vi "3phColor.vi"(4 "error in (no error)":errorcluster, 7 "Waveform Graph":refnum<vi>) -> (0 "error out":errorcluster)   [LabVIEW 2010]
panel:
  out "Array":u32[](array[numeric]) format="%06x"
  out "Label.Text":string
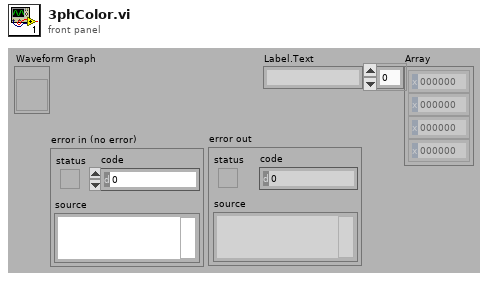
[diagram p1: front panel]
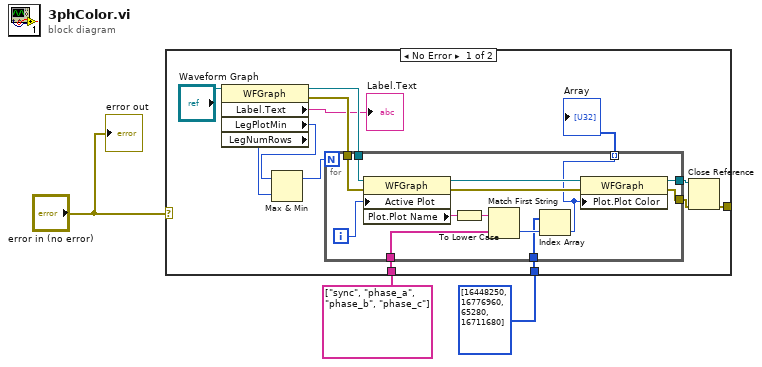
[diagram p0: block diagram]
diagram:
  n1 = case shown="No Error" "error in (no error)" {
    tunnel: [w11 _] -> _
    tunnel: string[] ["sync", "phase_a", "phase_b", "phase_c"] -> [w5 _]
    tunnel: u32[] [16448250, 16776960, 65280, 16711680] -> [w4 _]
    frame No Error {
      n2 = property on="Property Node" class="WFGraph"(reference="Waveform Graph") -> (reference out=w16:refnum<vi>, error out=w15:errorcluster, "Label.Text"=→"Label.Text":string, "LegPlotMin"=w8:u32, "LegNumRows"=w7:u32)  [unwired: 1 in]
      n3 = Max & Min(x=w8, y=w7) -> (max(x,y)=w6:u32)  [unwired: 1 out]
      n4 = for {
        N: w6 -> [_]
        tunnel: w16 -> [w28]
        tunnel: w15 -> [w26]
        tunnel: [w24] -> w13
        tunnel: [w23] -> w12
        tunnel: [w17] -> w9 mode=indexing
        tunnel: w5 -> [w19]
        tunnel: w4 -> [w18]
        i -> [w29]
        n5 = property on="Property Node" class="WFGraph"(reference=w28, error in=w26, "Active Plot"=w29) -> (reference out=w27:refnum<vi>, error out=w25:errorcluster, "Plot.Plot Name"=w22:string)
        n6 = To Lower Case(string=w22) -> (all lower case string=w21:string)
        n7 = Match First String(2:w19, 3:w21) -> (0:w20:i32)  [unwired: 1 out]
        n8 = Index Array(array=w18, index=w20) -> (element=w17:u32)
        n9 = property on="Property Node" class="WFGraph"(reference=w27, error in=w25, "Plot.Plot Color"=w17) -> (reference out=w24:refnum<vi>, error out=w23:errorcluster)
      }
      "Array" <- w9
      n10 = Close Reference(reference=w13, error in (no error)=w12) -> (error out=w11:errorcluster)
    }
    frame Error {
    }
  }
  "error out" <- "error in (no error)"
